vi "Get Parameter Definition.vi"(8 "error in":errorcluster, 11 "parameter ref in":T1 format="%.0x") -> (0 "error out":errorcluster, 2 "parameter definition":T2, 3 "parameter ref out":T1 format="%.0x")   [LabVIEW 2020, in "AIM ARINC 429 Scripting.lvlib"]
uses:
  AIM ARINC 429 Scripting.lvlib
  Shared/Parameter Definition.ctl
  <vilib>/NI/NI VeriStand Encoding and Decoding/Encoding.ctl
  <vilib>/NI VeriStand/Custom Device API/Custom Device Item Ref.ctl
  <vilib>/NI/NI VeriStand Encoding and Decoding/Encoding and Decoding.lvlib
  <vilib>/NI VeriStand/Custom Device API/Custom Device API.lvlib
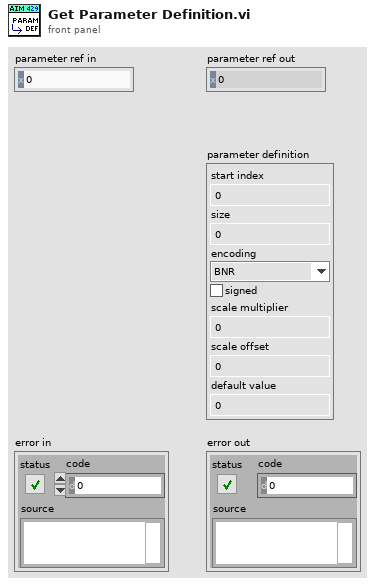
[diagram p1: front panel]
types:
  T1 = typedef "Custom Device API.lvlib/Custom Device Item Ref.ctl" = u64
  T2 = typedef "Parameter Definition.ctl" = cluster{"start index":i32, "size":i32, "encoding":T3, "signed":bool, "scale multiplier":dbl, "scale offset":dbl, "default value":dbl}
  T3 = typedef "Encoding and Decoding.lvlib/Encoding.ctl" = enum16{"BNR", "BCD", "Discrete"}
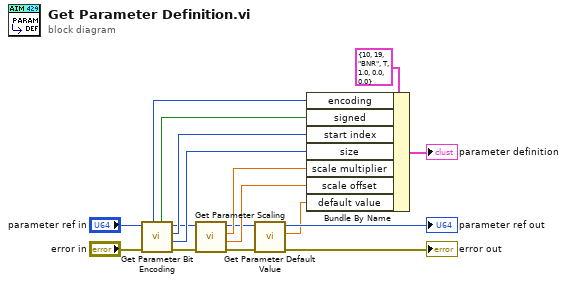
[diagram p0: block diagram]
diagram:
  n1 = call "Get Parameter Bit Encoding.vi"("error in"="error in", "parameter ref in"="parameter ref in") -> ("error out"=w9:errorcluster, "number of bits"=w14:i32, "start bit"=w13:i32, "parameter ref out"=w8:T1, "signed?"=w12:bool, "encoding type"=w11:T3)  [unwired: 4 in]
  n2 = call "Get Parameter Scaling.vi"("error in (no error)"=w9, "parameter ref in"=w8) -> ("error out"=w3:errorcluster, "scale offset"=w16:dbl, "scale multiplier"=w15:dbl, "parameter ref out"=w5:T1)  [unwired: 6 in]
  n3 = call "Get Parameter Default Value.vi"("error in"=w3, "parameter ref"=w5) -> ("error out"=→"error out":errorcluster, "Default Value (Scaled)"=w1:dbl, "parameter ref out"=→"parameter ref out":T1)  [unwired: 7 in]
  n4 = Bundle By Name(cluster=T2 {"start index"=10, "size"=19, "encoding"=enum."BNR", "signed"=TRUE, "scale multiplier"=1.0, "scale offset"=0.0, "default value"=0.0} ("parameter definition in"), "encoding"=w11, "signed"=w12, "start index"=w13, "size"=w14, "scale multiplier"=w15, "scale offset"=w16, "default value"=w1) -> (→"parameter definition":T2)
